vi "lsignKey.vi"(0 "MoAgSy_GPG":refnum<class "MoAgSy_GPG.lvclass">, 1 "options file":path, 2 "keyringfile":path, 3 "Sec keyringfile":path, 4 "id2sign":string, 5 "error in (no error)":errorcluster, 6 "key-id":string, 7 "password":string, 8 "Trust DB":path) -> (10 "dup Trust DB":path, 11 "standard output":string, 13 "data error?":bool, 14 "dup MoAgSy_GPG":refnum<class "MoAgSy_GPG.lvclass">, 15 "dup options file":path, 16 "dup keyringfile":path, 17 "dup Sec keyringfile":path, 18 "standard error":string, 19 "error out":errorcluster)   [LabVIEW 2009, in "MoAgSy.lvlib" / "MoAgSy_GPG.lvclass"]
doc: "Sign a GPG-Key for local use. This signature will not be exported with the key, or updated to a server."
uses:
  MoAgSy_GPG.lvclass
  HGF_GPG/HGF_GPG.lvclass/HGF_GPG.lvclass
panel:
  in  "Enum":T1(ring)
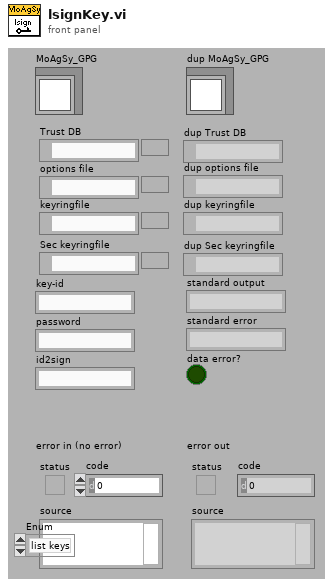
[diagram p1: front panel]
types:
  T1 = enum16{"list keys", "export", "import", "delete"}
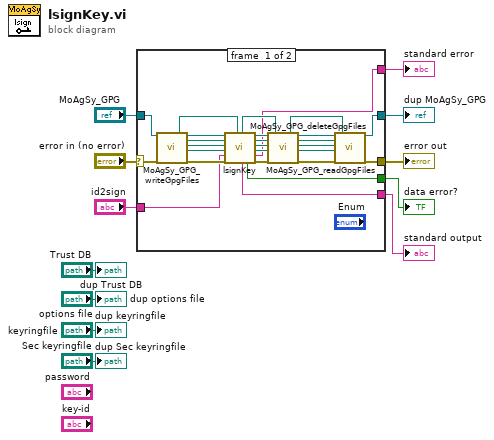
[diagram p0: block diagram]
diagram:
  n1 = case shown="No Error" "error in (no error)" {
    selector: "error in (no error)" -> [w13 w40]
    tunnel: [w38 w39] -> w7
    tunnel: [w37 w40] -> w1
    tunnel: "MoAgSy_GPG" -> [w30 w39]
    tunnel: "id2sign" -> [w17 _]
    tunnel: [w16 _] -> w5
    tunnel: [w15 _] -> w4
    tunnel: [w14 _] -> w3
    frame #0 {
      n2 = call "MoAgSy_GPG_writeGpgFiles.vi"("MoAgSy_GPG"=w30, "error in (no error)"=w13) -> ("trust db file"=w21:path, "dup MoAgSy_GPG"=w29:refnum<class "MoAgSy_GPG.lvclass">, "options file"=w25:path, "keyring file"=w26:path, "sec keyring file"=w27:path, "error out"=w19:errorcluster)  [unwired: 12 out]
      n3 = call-parent "lsignKey.vi"("HGF_GPG"=w29, "options file"=w25, "keyringfile"=w26, "Sec keyringfile"=w27, "id2sign"=w17, "error in (no error)"=w19, "Trust DB"=w21) -> ("dup Trust DB"=w20:path, "standard output"=w15:string, "data error?"=w14:bool, "dup HGF_GPG"=w28:refnum<class "MoAgSy_GPG.lvclass">, "dup options file"=w22:path, "dup keyringfile"=w23:path, "dup Sec keyringfile"=w24:path, "standard error"=w16:string, "error out"=w18:errorcluster)  [unwired: 4 in]
      n4 = call "MoAgSy_GPG_readGpgFiles.vi"("MoAgSy_GPG in"=w28, "options file"=w22, "keyring file"=w23, "sec keyring file"=w24, "error in (no error)"=w18, "trust db file"=w20) -> ("dup trust db file"=w35:path, "MoAgSy_GPG out"=w36:refnum<class "MoAgSy_GPG.lvclass">, "dup options file"=w34:path, "dup keyring file"=w33:path, "dup sec keyring file"=w32:path, "error out"=w31:errorcluster)  [unwired: 2 in, 6 out]
      n5 = call "MoAgSy_GPG_deleteGpgFiles.vi"("MoAgSy_GPG"=w36, "options file"=w34, "keyringfile"=w33, "Sec keyringfile"=w32, "error in (no error)"=w31, "Trust DB"=w35) -> ("dup MoAgSy_GPG"=w38:refnum<class "MoAgSy_GPG.lvclass">, "error out"=w37:errorcluster)  [unwired: 12 out]
    }
    frame #1 {
    }
  }
  "error out" <- w1
  "dup MoAgSy_GPG" <- w7
  "data error?" <- w3
  "standard output" <- w4
  "standard error" <- w5
  "dup options file" <- "options file"
  "dup keyringfile" <- "keyringfile"
  "dup Sec keyringfile" <- "Sec keyringfile"
  "dup Trust DB" <- "Trust DB"
